vi "Static String.vi"   [LabVIEW 2017, in "Memory Manager.lvlib" / "Static Error Handling.lvlib"]
uses:
  Static Error Handling.lvlib
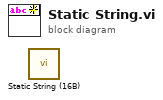
[diagram p0: block diagram]
diagram:
  n1 = call "Static String (16B).vi"() -> ()  [unwired: 11 in, 1 out]
